vi "CStoreSCU.vi"() -> ()   [LabVIEW 2013]
panel:
  out "return code":i32
  in  "port":string="11112"
  in  "server(ip)":string="www.dicomserver.co.uk "
  in  "aec":string="ANY-SCP"
  in  "aet":string="SCU"
  in  "standard input":string="-v -aet SCU -aec ANY-SCP www.dicomserver.co.uk 11112"
  in  "executable path":string="../DICOM/dcmtk/bin/echoscu.exe"
  in  "error in (no error)":errorcluster
  out "error out":errorcluster
  out "standard error":string
  out "standard output":string
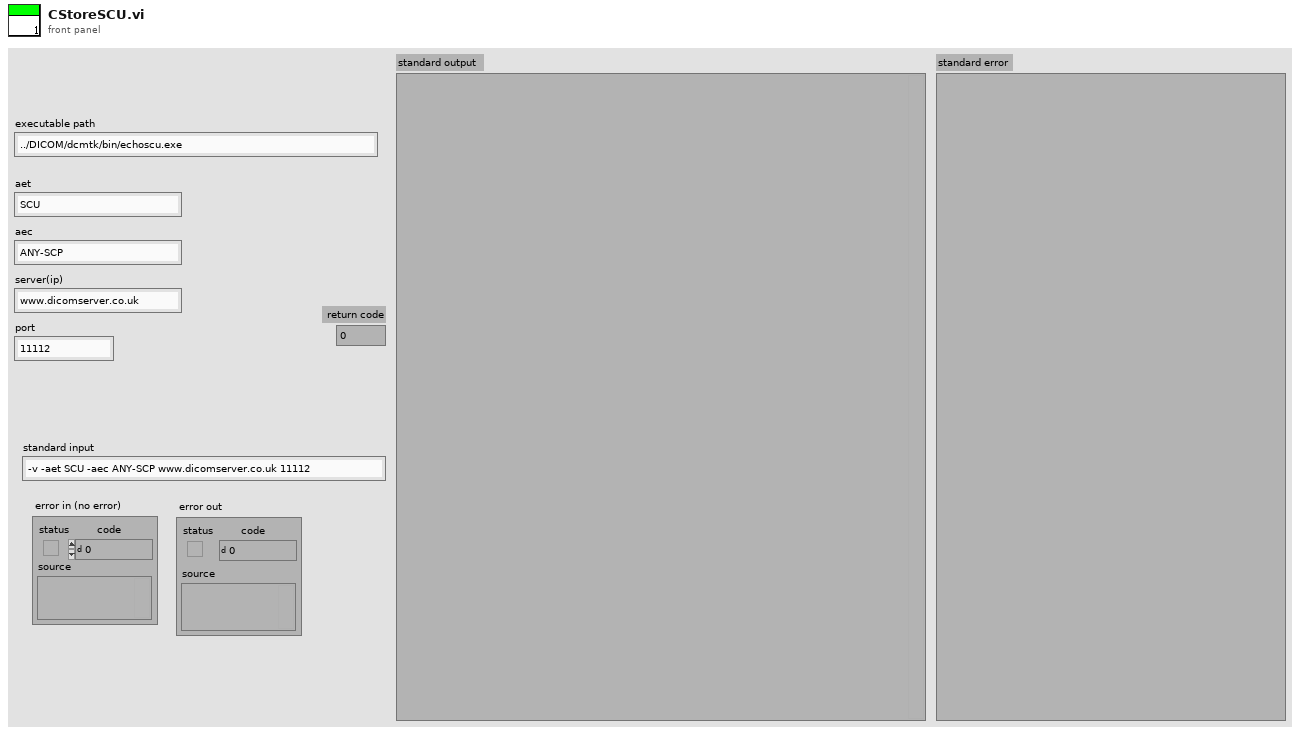
[diagram p1: front panel]
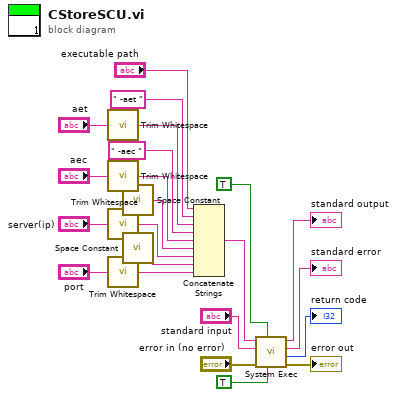
[diagram p0: block diagram]
diagram:
  n1 = call <vilib>:"Trim Whitespace.vi"("string"="aet") -> ("trimmed string"=w10:string)  [unwired: 1 in]
  n2 = call <vilib>:"Trim Whitespace.vi"("string"="aec") -> ("trimmed string"=w8:string)  [unwired: 1 in]
  n3 = call <vilib>:"Trim Whitespace.vi"("string"="server(ip)") -> ("trimmed string"=w2:string)  [unwired: 1 in]
  n4 = call <vilib>:"Trim Whitespace.vi"("string"="port") -> ("trimmed string"=w4:string)  [unwired: 1 in]
  n5 = call <vilib>:"Space Constant.vi"() -> ("String"=w7:string)
  n6 = call <vilib>:"Space Constant.vi"() -> ("String"=w6:string)
  n7 = Concatenate Strings("executable path", " -aet " ("string"), w10, " -aec " ("string"), w8, w7, w2, w6, w4) -> (w15:string)
  n8 = call <vilib>:"System Exec.vi"("run minimized? (F)"=TRUE, "wait until completion? (T)"=TRUE, "error in (no error)"="error in (no error)", "standard input"="standard input", "command line"=w15) -> ("error out"=→"error out":errorcluster, "return code"=→"return code":i32, "standard error"=→"standard error":string, "standard output"=→"standard output":string)  [unwired: 3 in]
